vi "Test App Error Handler is Configured for Process Added after Setting Error Handler.vi"(8 "error in (no error)":errorcluster, 11 "Rig Test In":refnum<class "Application Test.lvclass">) -> (0 "error out":errorcluster, 3 "Rig Test Out":refnum<class "Application Test.lvclass">)   [LabVIEW 2020, in "Application Test.lvclass"]
uses:
  Application Test.lvclass
  C:/Program Files (x86)/National Instruments/LabVIEW 2020/vi.lib/Asteme/LUnit/Test Case.lvclass
  Mock Error Handler/Mock Error Handler.lvclass
  C:/Users/anton/Documents/GitHub/Triarc-Framework/source/Framework/Error Handler Interface/Error Handler Interface.lvclass
  Mock Process/Mock Process.lvclass
  C:/Users/anton/Documents/GitHub/Triarc-Framework/source/Framework/Process/Process.lvclass
  Framework/Process/Process.lvclass/Process.ctl
  Framework/Application/Application.lvclass/Application.ctl
  <vilib>/Asteme/LUnit/Test Case.lvclass/Test Case.ctl
  <vilib>/Asteme/LUnit/LUnit Assertion Result.lvclass/LUnit Assertion Result.ctl
  Framework/Process/Public/Lifecycle/Get Lifecycle State.vi
  Framework/Process/Protected/Messaging/Enqueue Message.vi
  <vilib>/Utility/error.llb/Clear Errors.vi
  Framework/Application/Private/Add Process to Map.vi
  Framework/Process/Protected/SubVIs/Set Context.vi
  Framework/Process/Private/SubVIs/Wait for finish.vi
  Framework/Process/Private/SubVIs/Set Lifecycle State.vi
  Framework/Process/Protected/Messaging/Request Message.vi
  <vilib>/Asteme/LUnit/Palette/Pass.vi
  <vilib>/Asteme/LUnit/Palette/Fail.vi
  <vilib>/Asteme/LUnit/Variant to string.vi
  <vilib>/Asteme/LUnit/Set Assertion Type.vi
  <vilib>/AdvancedString/1D String Array to Delimited String.vi
  Framework/Process/Community/Leave Process Loop.vi
  Framework/Process/Private/SubVIs/Enqueue Request Message.vi
  <vilib>/Asteme/LUnit/Add test result.vi
  <vilib>/Asteme/LUnit/LUnit Write Passed.vi
  <vilib>/Asteme/LUnit/LUnit Get Test Case.vi
  <vilib>/Asteme/LUnit/LUnit Write Message.vi
  <vilib>/Asteme/LUnit/LUnit Write Description.vi
  <vilib>/Asteme/LUnit/LUnit Write Assertion Type.vi
  <vilib>/Asteme/LUnit/Read Test Case Name.vi
  Framework/Application/Application.lvclass
  <vilib>/Utility/error.llb/Error Cluster From Error Code.vi
  Framework/Process/Private/SubVIs/Wait for Response Message.vi
  <vilib>/Asteme/LUnit/Assertion Result/LUnit Get Test Name.vi
  <vilib>/Utility/Data Type/Get Type Information.vi
  <vilib>/Utility/LVClass/Get LV Class Name.vi
  Framework/Process/Process.lvclass
  <vilib>/Asteme/LUnit/LUnit Assertion Result.lvclass
  <vilib>/Asteme/LUnit/Test Case.lvclass
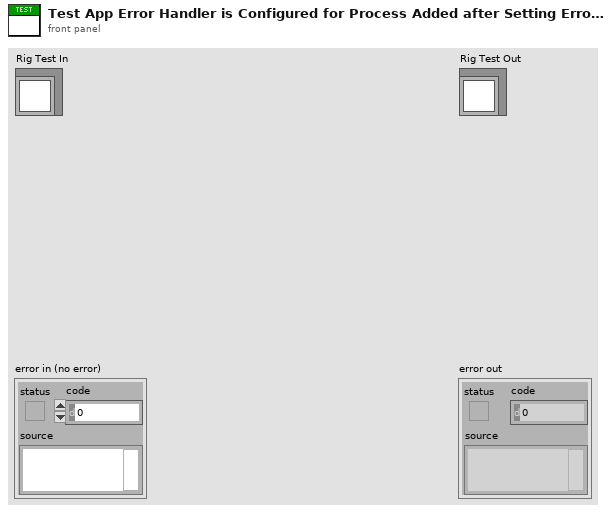
[diagram p1: front panel]
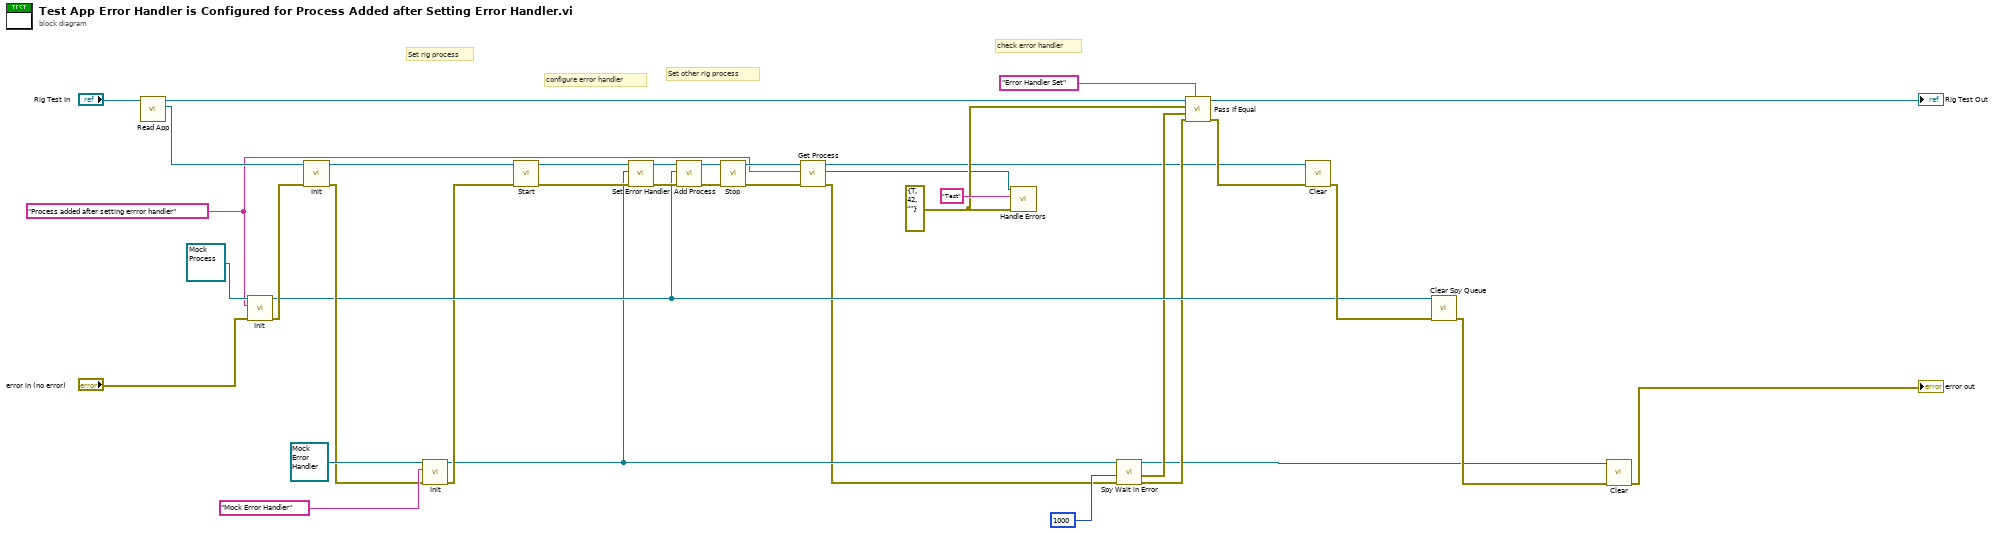
[diagram p0: block diagram]
diagram:
  w11 = errorcluster {"status"=TRUE, "code"=42, "source"=""} ("error in (no error)")
  w2 = "Process added after setting errror handler" ("Name")
  # "check error handler"
  # "Set other rig process"
  # "configure error handler"
  # "Set rig process"
  n1 = call "Read App.vi"("Application Test In"="Rig Test In") -> ("App out"=w36:refnum<class "Application.lvclass">, "Application Test Out"=w32:refnum<class "Application Test.lvclass">)  [unwired: 8 in, 1 out]
  n2 = call-dynamic "Init.vi"("error in (no error)"="error in (no error)", "Name"=w2, "Mock Process In"=refnum<class "Mock Process.lvclass"> refnum ("Mock Process.lvclass")) -> ("error out"=w27:errorcluster, "Mock Process Out"=w14:refnum<class "Mock Process.lvclass">)  [unwired: 7 in]
  n3 = call-dynamic "Init.vi"("error in (no error)"=w27, "Process In"=w36) -> ("error out"=w26:errorcluster, "Process Out"=w35:refnum<class "Application.lvclass">)  [unwired: 8 in]
  n4 = call-dynamic "Init.vi"("error in (no error)"=w26, "Name"="Mock Error Handler", "Mock Error Handler In"=refnum<class "Mock Error Handler.lvclass"> refnum ("Mock Error Handler.lvclass")) -> ("error out"=w9:errorcluster, "Mock Error Handler Out"=w8:refnum<class "Mock Error Handler.lvclass">)  [unwired: 7 in]
  n5 = call "Start.vi"("error in (no error)"=w9, "Process In"=w35) -> ("error out"=w21:errorcluster, "Process Out"=w22:refnum<class "Application.lvclass">)  [unwired: 8 in]
  n6 = call "Set Error Handler.vi"("error in (no error)"=w21, "Error Handler"=w8, "Process In"=w22) -> ("error out"=w17:errorcluster, "Process Out"=w18:refnum<class "Application.lvclass">)  [unwired: 7 in]
  n7 = call "Add Process.vi"("error in (no error)"=w17, "Process"=w14, "Rig In"=w18) -> ("error out"=w15:errorcluster, "Rig Out"=w16:refnum<class "Application.lvclass">)  [unwired: 7 in]
  n8 = call "Stop.vi"("error in (no error)"=w15, "Process In"=w16) -> ("error out"=w23:errorcluster, "Process Out"=w4:refnum<class "Application.lvclass">)  [unwired: 7 in, 1 out]
  n9 = call "Get Process.vi"("error in (no error)"=w23, "Process Name"=w2, "Rig In"=w4) -> ("error out"=w5:errorcluster, "App Process"=w1:refnum<class "Process.lvclass">, "Rig Out"=w3:refnum<class "Application.lvclass">)  [unwired: 6 in]
  n10 = call-dynamic "Handle Errors.vi"("error in (no error)"=w11, "Location"="Test", "Process In"=w1) -> ()  [unwired: 7 in, 2 out]
  n11 = call "Spy Wait in Error.vi"("error in (no error)"=w5, "timeout in ms (-1)"=1000, "Mock Error Handler In"=w8) -> ("error out"=w12:errorcluster, "Errors"=w10:errorcluster, "Mock Error Handler Out"=w7:refnum<class "Mock Error Handler.lvclass">)  [unwired: 4 in, 2 out]
  n12 = call <vilib>:"Pass If Equal.vi"("Description"="Error Handler Set", "error in (no error)"=w12, "Actual"=w10, "Expected"=w11, "Test Case In"=w32) -> ("error out"=w25:errorcluster, "Test Case Out"=→"Rig Test Out":refnum<class "Application Test.lvclass">)  [unwired: 5 in]
  n13 = call-dynamic "Clear.vi"("error in (no error)"=w25, "Application In"=w3) -> ("error out"=w20:errorcluster)  [unwired: 8 in, 1 out]
  n14 = call-dynamic "Clear Spy Queue.vi"("error in (no error)"=w20, "Mock Process In"=w14) -> ("error out"=w19:errorcluster)  [unwired: 8 in, 1 out]
  n15 = call-dynamic "Clear.vi"("error in (no error)"=w19, "Mock Process In"=w7) -> ("error out"=→"error out":errorcluster)  [unwired: 8 in, 1 out]
